vi "Extended User Data.vi"(7 "Action (1: Write Data)":i32(ring)=1 items=["Read Data", "Write Data", "Clear Data", "Clear ALL Data"], 8 "error in (no error)":errorcluster, 10 "User Data In":T1={"X-Series Mode"=97, "Acquisition Type (0: Normal)"=0} {"Acquisition Type (0: Normal)" items=["Normal", "Average", "High Resolution", "Peak"]; "X-Series Mode" items=["MSO-X 3014A", "MSO-X 3024A", "MSO-X 3034A", "MSO-X 3054A", "MSO-X 3012A", "MSO-X 3022A", "MSO-X 3032A", "MSO-X 3052A", "MSO-X 2004A", "MSO-X 2014A", "MSO-X 2024A", "MSO-X 2002A", "MSO-X 2012A", "MSO-X 2022A", "MSO-X 3104A", "MSO-X 3102A", "MSO-X 4154A", "MSO-X 4104A", "MSO-X 4054A", "MSO-X 4034A", "MSO-X 4024A", "MSO-X 4052A", "MSO-X 4032A", "MSO-X 4022A", "DSO-X 3014A", "DSO-X 3024A", "DSO-X 3034A", "DSO-X 3054A", "DSO-X 3012A", "DSO-X 3022A", "DSO-X 3032A", "DSO-X 3052A", "DSO-X 2004A", "DSO-X 2014A", "DSO-X 2024A", "DSO-X 2002A", "DSO-X 2012A", "DSO-X 2022A", "DSO-X 3104A", "DSO-X 3102A", "DSO-X 4154A", "DSO-X 4104A", "DSO-X 4054A", "DSO-X 4034A", "DSO-X 4024A", "DSO-X 4052A", "DSO-X 4032A", "DSO-X 4022A", "DSO-X 3012T", "DSO-X 3014T", "DSO-X 3022T", "DSO-X 3024T", "DSO-X 3032T", "DSO-X 3034T", "DSO-X 3052T", "DSO-X 3054T", "DSO-X 3102T", "DSO-X 3104T", "MSO-X 3012T", "MSO-X 3014T", "MSO-X 3022T", "MSO-X 3024T", "MSO-X 3032T", "MSO-X 3034T", "MSO-X 3052T", "MSO-X 3054T", "MSO-X 3102T", "MSO-X 3104T", "DSO-X 6002A", "DSO-X 6004A", "MSO-X 6002A", "MSO-X 6004A", "EDU-X 1002A", "EDU-X 1002G", "DSO-X 1102A", "DSO-X 1102G", "EDUX1052A", "EDUX1052G", "DSOX1202A", "DSOX1202G", "DSOX1204A", "DSOX1204G", "DSO-X 3012G", "DSO-X 3014G", "DSO-X 3022G", "DSO-X 3024G", "DSO-X 3032G", "DSO-X 3034G", "DSO-X 3052G", "DSO-X 3054G", "DSO-X 30102G", "DSO-X 30104G", "MSO-X 3012G", "MSO-X 3014G", "MSO-X 3022G", "MSO-X 3024G", "MSO-X 3032G", "MSO-X 3034G", "MSO-X 3052G", "MSO-X 3054G", "MSO-X 30102G", "MSO-X 30104G", "EL34243A"]}, 11 "VISA resource name in":refnum<visa-resource-name>="MSOX3054") -> (0 "error out":errorcluster, 2 "User Data Out":T1 {"Acquisition Type (0: Normal)" items=["Normal", "Average", "High Resolution", "Peak"]; "X-Series Mode" items=["MSO-X 3014A", "MSO-X 3024A", "MSO-X 3034A", "MSO-X 3054A", "MSO-X 3012A", "MSO-X 3022A", "MSO-X 3032A", "MSO-X 3052A", "MSO-X 2004A", "MSO-X 2014A", "MSO-X 2024A", "MSO-X 2002A", "MSO-X 2012A", "MSO-X 2022A", "MSO-X 3104A", "MSO-X 3102A", "MSO-X 4154A", "MSO-X 4104A", "MSO-X 4054A", "MSO-X 4034A", "MSO-X 4024A", "MSO-X 4052A", "MSO-X 4032A", "MSO-X 4022A", "DSO-X 3014A", "DSO-X 3024A", "DSO-X 3034A", "DSO-X 3054A", "DSO-X 3012A", "DSO-X 3022A", "DSO-X 3032A", "DSO-X 3052A", "DSO-X 2004A", "DSO-X 2014A", "DSO-X 2024A", "DSO-X 2002A", "DSO-X 2012A", "DSO-X 2022A", "DSO-X 3104A", "DSO-X 3102A", "DSO-X 4154A", "DSO-X 4104A", "DSO-X 4054A", "DSO-X 4034A", "DSO-X 4024A", "DSO-X 4052A", "DSO-X 4032A", "DSO-X 4022A", "DSO-X 3012T", "DSO-X 3014T", "DSO-X 3022T", "DSO-X 3024T", "DSO-X 3032T", "DSO-X 3034T", "DSO-X 3052T", "DSO-X 3054T", "DSO-X 3102T", "DSO-X 3104T", "MSO-X 3012T", "MSO-X 3014T", "MSO-X 3022T", "MSO-X 3024T", "MSO-X 3032T", "MSO-X 3034T", "MSO-X 3052T", "MSO-X 3054T", "MSO-X 3102T", "MSO-X 3104T", "DSO-X 6002A", "DSO-X 6004A", "MSO-X 6002A", "MSO-X 6004A", "EDU-X 1002A", "EDU-X 1002G", "DSO-X 1102A", "DSO-X 1102G", "EDUX1052A", "EDUX1052G", "DSOX1202A", "DSOX1202G", "DSOX1204A", "DSOX1204G", "DSO-X 3012G", "DSO-X 3014G", "DSO-X 3022G", "DSO-X 3024G", "DSO-X 3032G", "DSO-X 3034G", "DSO-X 3052G", "DSO-X 3054G", "DSO-X 30102G", "DSO-X 30104G", "MSO-X 3012G", "MSO-X 3014G", "MSO-X 3022G", "MSO-X 3024G", "MSO-X 3032G", "MSO-X 3034G", "MSO-X 3052G", "MSO-X 3054G", "MSO-X 30102G", "MSO-X 30104G", "EL34243A"]}, 3 "VISA resource name out":refnum<visa-resource-name>="MSOX3054")   [LabVIEW 2015, in "Agilent 2000 3000 X-Series.lvlib"]
doc: "You can use this vi to perform an action on current VI settings, such as write, read, clear and clear all."
uses:
  Agilent 2000 3000 X-Series.lvlib
  Extended User Data.ctl
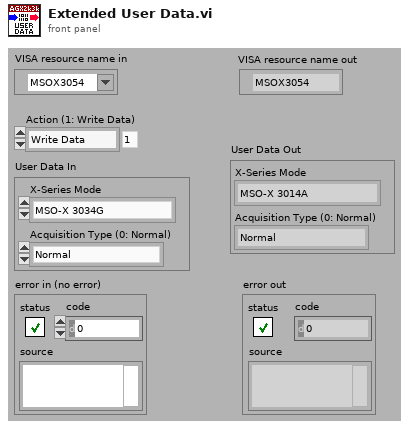
[diagram p1: front panel]
types:
  T1 = typedef "Agilent 2000 3000 X-Series.lvlib/Extended User Data.ctl" = cluster{"X-Series Mode":u16, "Acquisition Type (0: Normal)":i32}
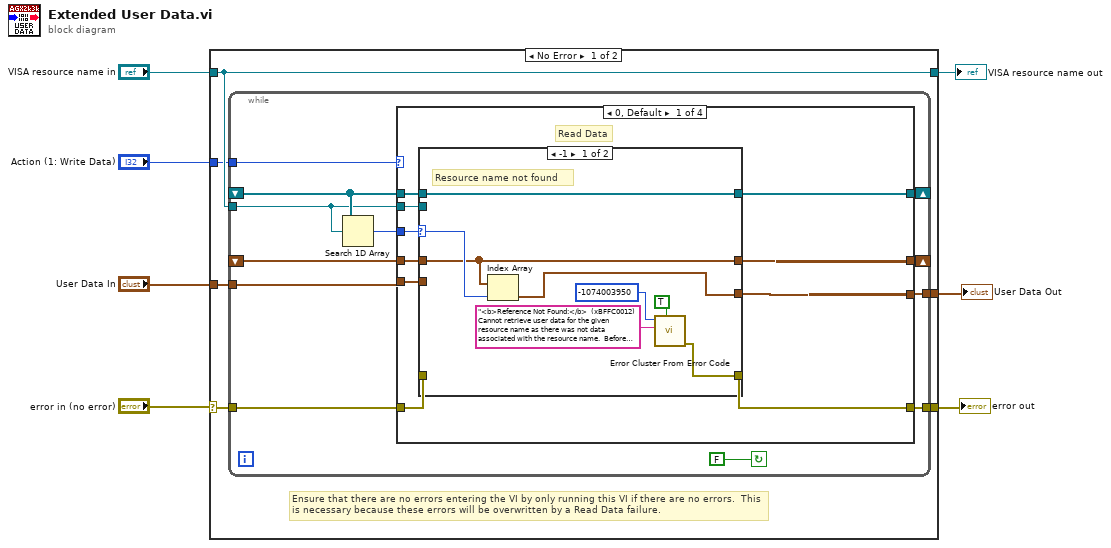
[diagram p0: block diagram]
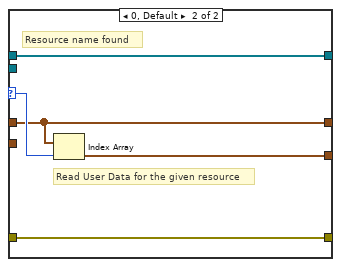
[diagram p2: hidden frame]
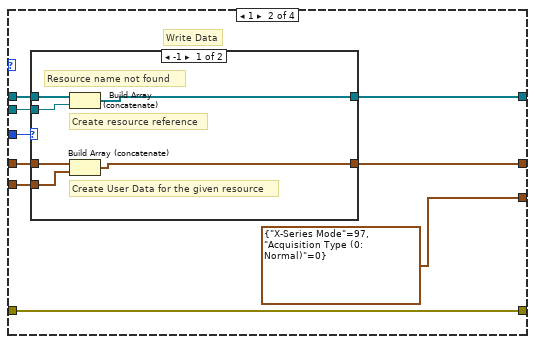
[diagram p3: hidden frame]
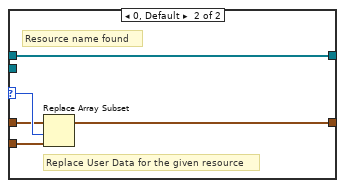
[diagram p4: hidden frame]
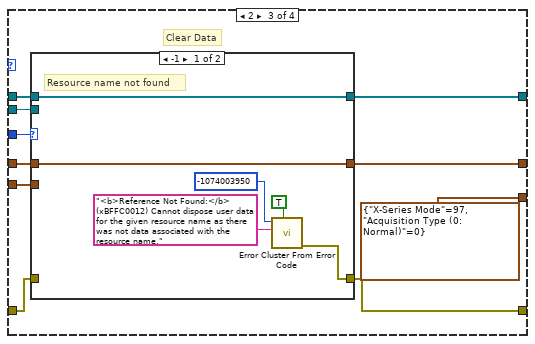
[diagram p5: hidden frame]
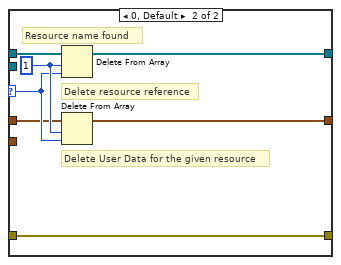
[diagram p6: hidden frame]
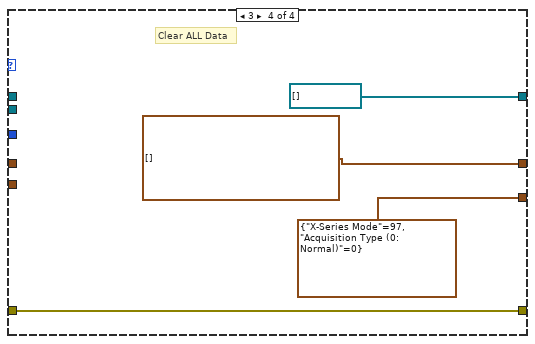
[diagram p7: hidden frame]
diagram:
  n1 = case shown="No Error" "error in (no error)" {
    selector: "error in (no error)" -> [w12 w98]
    tunnel: "VISA resource name in" -> [w11 w97]
    tunnel: [w13 w98] -> w5
    tunnel: [w11 w97] -> w4
    tunnel: "User Data In" -> [w10 w96]
    tunnel: [w9 w96] -> w2
    tunnel: "Action (1: Write Data)" -> [w8 _]
    frame No Error {
      # "Ensure that there are no errors entering the VI by only running this VI if there are no errors.  This is necessary because these errors will be overwritten by a Read Data failure."
      n2 = while {
        shift-right: [w23] -> _
        shift-left: _ -> [w24]
        tunnel: w11 -> [w22]
        tunnel: w12 -> [w20]
        tunnel: [w19] -> w13
        shift-right: [w18] -> _
        shift-left: _ -> [w17]
        tunnel: w10 -> [w16]
        tunnel: [w15] -> w9
        tunnel: w8 -> [w14]
        stop <- FALSE continue-if-true
        n3 = Search 1D Array(1D array=w24, element=w22) -> (index of element=w25:i32)  [unwired: 1 out]
        n4 = case shown="0, Default" w14 {
          tunnel: w16 -> [w35 w57 w78 _]
          tunnel: w25 -> [w34 w56 w77 _]
          tunnel: w24 -> [w33 w55 w76 _]
          tunnel: [w32 w54 w75 refnum<visa-resource-name>[] []] -> w23
          tunnel: w22 -> [w31 w53 w74 _]
          tunnel: w20 -> [w29 w52 w72 w94]
          tunnel: [w30 w52 w73 w94] -> w19
          tunnel: [w28 w51 w70 T1[] []] -> w18
          tunnel: w17 -> [w27 w50 w71 _]
          tunnel: [w26 T1 {"X-Series Mode"=97, "Acquisition Type (0: Normal)"=0} ("User Data In") T1 {"X-Series Mode"=97, "Acquisition Type (0: Normal)"=0} ("User Data In") T1 {"X-Series Mode"=97, "Acquisition Type (0: Normal)"=0} ("User Data In")] -> w15
          frame 0, Default {
            # "Read Data"
            n5 = case shown="-1" w34 {
              selector: w34 -> [w38 w48]
              tunnel: w35 -> [_ _]
              tunnel: w33 -> [w43 w47]
              tunnel: [w43 w47] -> w32
              tunnel: w31 -> [_ _]
              tunnel: [w42 w46] -> w30
              tunnel: w29 -> [_ w46]
              tunnel: [w37 w45] -> w28
              tunnel: w27 -> [w37 w45]
              tunnel: [w36 w44] -> w26
              frame -1 {
                # "Resource name not found"
                n6 = Index Array(array=w37, index=w38) -> (element=w36:T1)
                n7 = call <vilib>:"Error Cluster From Error Code.vi"("show call chain? (False)"=TRUE, "error message (\"\")"="<b>Reference Not Found:</b>  (xBFFC0012) Cannot retrieve user data for the given resource name as there was not data associated with the resource name.  Before you can read data, you need to write the user data using the Write Data action of this User Data VI. ", "error code (0)"=-1074003950 ("Code")) -> ("error out"=w42:errorcluster)  [unwired: 1 in, 5 out]
              }
              frame 0, Default {
                # "Read User Data for the given resource"
                # "Resource name found"
                n8 = Index Array(array=w45, index=w48) -> (element=w44:T1)
              }
            }
          }
          frame 1 {
            # "Write Data"
            n9 = case shown="-1" w56 {
              selector: w56 -> [_ w67]
              tunnel: w57 -> [w62 w68]
              tunnel: w55 -> [w63 w66]
              tunnel: [w60 w66] -> w54
              tunnel: w53 -> [w61 _]
              tunnel: [w59 w65] -> w51
              tunnel: w50 -> [w58 w64]
              frame -1 {
                # "Create resource reference"
                # "Create User Data for the given resource"
                # "Resource name not found"
                n10 = Build Array (concatenate)(w63, w61) -> (w60:refnum<visa-resource-name>[])
                n11 = Build Array (concatenate)(w58, w62) -> (w59:T1[])
              }
              frame 0, Default {
                # "Replace User Data for the given resource"
                # "Resource name found"
                n12 = Replace Array Subset(array=w64, new element=w68, index=w67) -> (w65:T1[])
              }
            }
          }
          frame 2 {
            # "Clear Data"
            n13 = case shown="-1" w77 {
              selector: w77 -> [_ w86]
              tunnel: w78 -> [_ _]
              tunnel: [w79 w91] -> w70
              tunnel: w76 -> [w84 w89]
              tunnel: [w84 w88] -> w75
              tunnel: w74 -> [_ _]
              tunnel: [w83 w90] -> w73
              tunnel: w72 -> [_ w90]
              tunnel: w71 -> [w79 w85]
              frame -1 {
                # "Resource name not found"
                n14 = call <vilib>:"Error Cluster From Error Code.vi"("show call chain? (False)"=TRUE, "error message (\"\")"="<b>Reference Not Found:</b>  (xBFFC0012) Cannot dispose user data for the given resource name as there was not data associated with the resource name.", "error code (0)"=-1074003950 ("Code")) -> ("error out"=w83:errorcluster)  [unwired: 1 in, 5 out]
              }
              frame 0, Default {
                w87 = 1 ("length")
                # "Delete resource reference"
                # "Delete User Data for the given resource"
                # "Resource name found"
                n15 = Delete From Array(array=w89, length=w87, index=w86) -> (array with subset deleted=w88:refnum<visa-resource-name>[])  [unwired: 1 out]
                n16 = Delete From Array(array=w85, length=w87, index=w86) -> (array with subset deleted=w91:T1[])  [unwired: 1 out]
              }
            }
          }
          frame 3 {
            # "Clear ALL Data"
          }
        }
      }
    }
    frame Error {
    }
  }
  "VISA resource name out" <- w4
  "error out" <- w5
  "User Data Out" <- w2
